vi "format time SDI data into XY plot input.vi"(9 "Measurement Array":dbl[][](array[numeric]), 10 "disabled index (col)":i32, 11 "Time Array":dbl[](array[numeric])) -> (3 "XY Graph":cluster{"X":dbl[], "Y":dbl[]}[](array[cluster]))   [LabVIEW 2016]
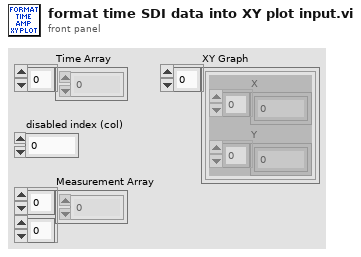
[diagram p1: front panel]
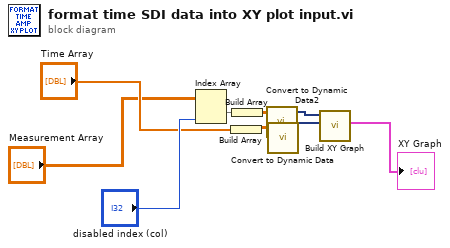
[diagram p0: block diagram]
diagram:
  n1 = Index Array(array="Measurement Array", index (col)="disabled index (col)") -> (element=w7:dbl[])  [unwired: 1 in]
  n2 = Build Array("Time Array") -> (w5:dbl[][])
  n3 = Build Array(w7) -> (w8:dbl[][])
  n4 = call "Convert to Dynamic Data2"("2D Array"=w8) -> ("Dynamic Data Type"=w2:dynamicdata)  [unwired: 3 in]
  n5 = call "Convert to Dynamic Data"("2D Array"=w5) -> ("Dynamic Data Type"=w3:dynamicdata)  [unwired: 3 in]
  n6 = call "Build XY Graph"("Y Input"=w3, "X Input"=w2) -> ("XY Graph"=→"XY Graph":cluster{"X":dbl[], "Y":dbl[]}[])  [unwired: 8 in, 1 out]
